vi "_RT_CtrlLoop_D999_Conv_Cmd.vi"(2 "error in (no error)":errorcluster, 3 "Head+Addr+Seg":string, 4 "CmdParam":T1={"Cmd"=enum."Init", "Variant"=variant}) -> (0 "error out":errorcluster, 1 "Cmd_String":string)   [LabVIEW 2018]
uses:
  PublicSubVI/Ctl/_ctl_RT_D999_Settings.ctl
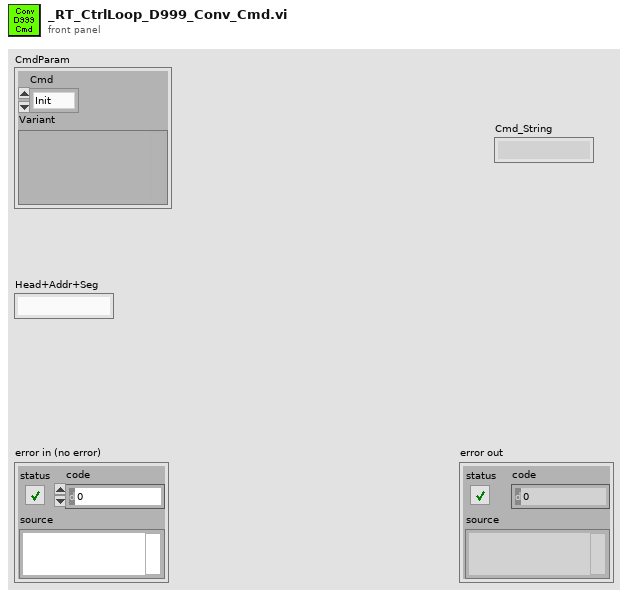
[diagram p1: front panel]
types:
  T1 = typedef "_ctl_RT_D999_Settings.ctl" = cluster{"Cmd":enum16{"None", "Init", "Write", "WriteAll", "Read", "ReadAll", "SetEnable", "SetParam", "ReadAO", "ReadSwitch", "ReportID"}, "Variant":variant}
  T2 = enum16{"None", "Init", "Write", "WriteAll", "Read", "ReadAll", "SetEnable", "SetParam", "ReadAO", "ReadSwitch", "ReportID"}
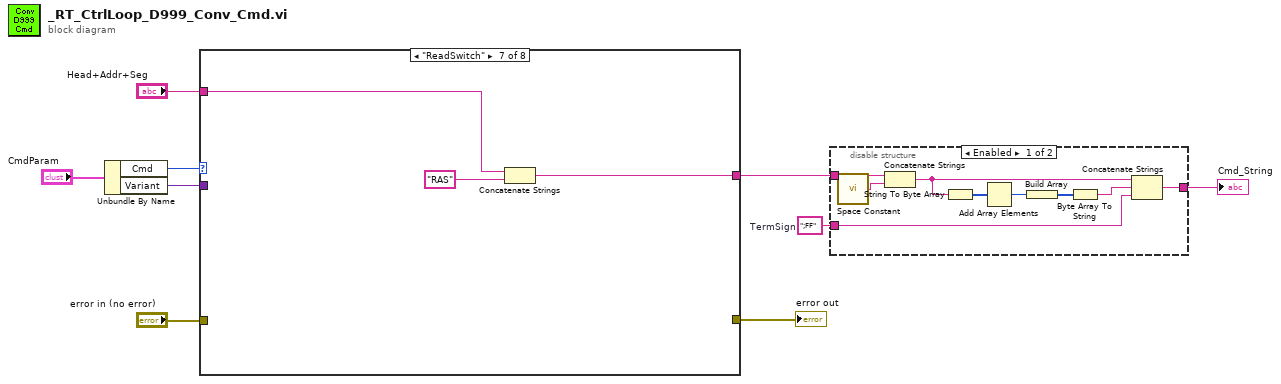
[diagram p0: block diagram]
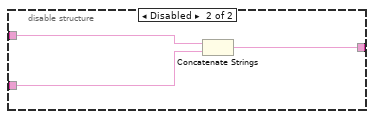
[diagram p2: hidden frame]
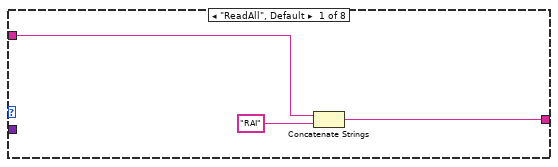
[diagram p3: hidden frame]
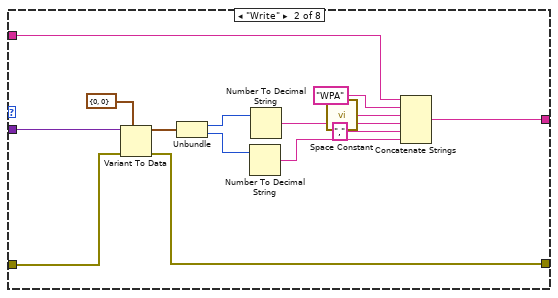
[diagram p4: hidden frame]
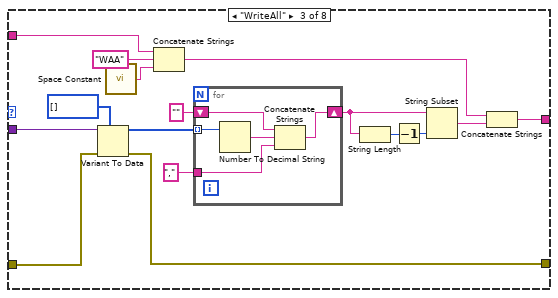
[diagram p5: hidden frame]
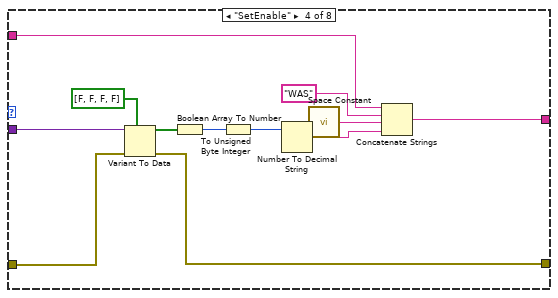
[diagram p6: hidden frame]
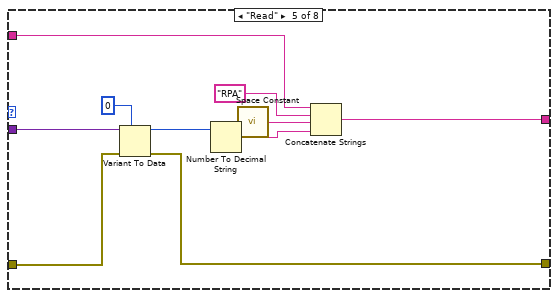
[diagram p7: hidden frame]
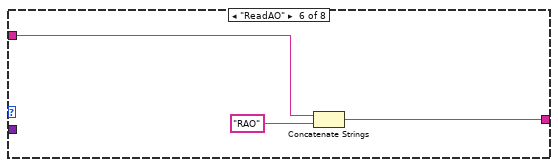
[diagram p8: hidden frame]
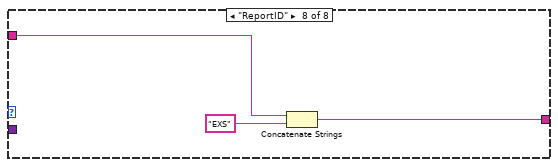
[diagram p9: hidden frame]
diagram:
  w1 = ";FF"  # TermSign
  n1 = Unbundle By Name("CmdParam") -> ("Cmd"=w8:T2, "Variant"=w7:variant)
  n2 = case shown="\"ReadSwitch\"" w8 {
    tunnel: w7 -> [_ w22 w30 w58 w68 _ _ _]
    tunnel: "Head+Addr+Seg" -> [w11 w18 w31 w56 w64 w71 w74 w78]
    tunnel: [w10 w19 w27 w57 w65 w70 w73 w76] -> w3
    tunnel: "error in (no error)" -> [_ w17 w29 w53 w61 _ _ _]
    tunnel: [_ w16 w28 w52 w60 _ _ _] -> w5
    frame "ReadAll", Default {
      n3 = Concatenate Strings(w11, "RAI" ("string")) -> (w10:string)
    }
    frame "Write" {
      n4 = Variant To Data(error in=w17, type=cluster{"Port":u8, "Value":i16} {"Port"=0, "Value"=0}, Variant=w22) -> (data=w21:cluster{"Port":u8, "Value":i16}, error out=w16:errorcluster)
      n5 = Unbundle(w21) -> ("Port"=w20:u8, "Value"=w15:i16)
      n6 = Number To Decimal String(number=w15) -> (decimal integer string=w14:string)  [unwired: 1 in]
      n7 = Number To Decimal String(number=w20) -> (decimal integer string=w24:string)  [unwired: 1 in]
      n8 = call <vilib>:"Space Constant.vi"() -> ("String"=w25:string)
      n9 = Concatenate Strings(w18, "WPA" ("string"), w25, w24, "," ("string"), w14) -> (w19:string)
    }
    frame "WriteAll" {
      n10 = Variant To Data(error in=w29, type=i32[] [] ("appended array"), Variant=w30) -> (data=w39:i32[], error out=w28:errorcluster)
      n11 = call <vilib>:"Space Constant.vi"() -> ("String"=w41:string)
      n12 = Concatenate Strings(w31, "WAA" ("string"), w41) -> (w33:string)
      n13 = for {
        tunnel: w39 -> [w47] mode=indexing
        tunnel: "," -> [w45]
        shift-right: [w44] -> w34
        shift-left: "" -> [w43]
        n14 = Number To Decimal String(number=w47) -> (decimal integer string=w46:string)  [unwired: 1 in]
        n15 = Concatenate Strings(w43, w46, w45) -> (w44:string)
      }
      n16 = String Length(string=w34) -> (length=w35:i32)
      n17 = Decrement(x=w35) -> (x-1=w36:i32)
      n18 = String Subset(string=w34, length (rest)=w36) -> (substring=w32:string)  [unwired: 1 in]
      n19 = Concatenate Strings(w33, w32) -> (w27:string)
    }
    frame "SetEnable" {
      n20 = Variant To Data(error in=w53, type=bool[] [FALSE, FALSE, FALSE, FALSE], Variant=w58) -> (data=w50:bool[], error out=w52:errorcluster)
      n21 = Boolean Array To Number(Boolean array=w50) -> (number=w49:u32)
      n22 = To Unsigned Byte Integer(number=w49) -> (unsigned 8bit integer=w48:u8)
      n23 = Number To Decimal String(number=w48) -> (decimal integer string=w54:string)  [unwired: 1 in]
      n24 = call <vilib>:"Space Constant.vi"() -> ("String"=w55:string)
      n25 = Concatenate Strings(w56, "WAS" ("string"), w55, w54) -> (w57:string)
    }
    frame "Read" {
      n26 = Variant To Data(error in=w61, type=0 ("number"), Variant=w68) -> (data=w66:i32, error out=w60:errorcluster)
      n27 = Number To Decimal String(number=w66) -> (decimal integer string=w62:string)  [unwired: 1 in]
      n28 = call <vilib>:"Space Constant.vi"() -> ("String"=w63:string)
      n29 = Concatenate Strings(w64, "RPA" ("string"), w63, w62) -> (w65:string)
    }
    frame "ReadAO" {
      n30 = Concatenate Strings(w71, "RAO" ("string")) -> (w70:string)
    }
    frame "ReadSwitch" {
      n31 = Concatenate Strings(w74, "RAS" ("string")) -> (w73:string)
    }
    frame "ReportID" {
      n32 = Concatenate Strings(w78, "EXS" ("string")) -> (w76:string)
    }
  }
  "error out" <- w5
  n33 = disable-structure shown="Enabled" {
    disable-tunnel: w3 -> [w84 w90]
    disable-tunnel: [w80 w88] -> w2
    disable-tunnel: w1 -> [w79 w89]
    frame Enabled {
      n34 = call <vilib>:"Space Constant.vi"() -> ("String"=w83:string)
      n35 = Concatenate Strings(w84, w83) -> (w82:string)
      n36 = String To Byte Array(string=w82) -> (unsigned byte array=w85:u8[])
      n37 = Add Array Elements(numeric array=w85) -> (sum=w87:u8)
      n38 = Build Array(w87) -> (w86:u8[])
      n39 = Byte Array To String(unsigned byte array=w86) -> (string=w81:string)
      n40 = Concatenate Strings(w82, w81, w79) -> (w80:string)
    }
    frame Disabled {
      n41 = Concatenate Strings(w90, w89) -> (w88:string)
    }
  }
  "Cmd_String" <- w2
